vi "Main.vi"() -> ()   [LabVIEW 2014]
uses:
  Tasks.ctl
  <vilib>/Platform/TimedLoop/XDataNode/timing_clust.ctl
  <vilib>/Platform/TimedLoop/XDataNode/nitl_modes.ctl
  <vilib>/Platform/TimedLoop/XDataNode/wakeup.ctl
  <vilib>/myRIO/Instrument Drivers/Onboard IO/AI/typedefs/AI Reference.ctl
  <vilib>/myRIO/Common/Instrument Driver Framework/Utilities/typedefs/myRIO Generic Hardware Reference.ctl
  <vilib>/myRIO/Common/Instrument Driver Framework/Utilities/typedefs/Hardware Version Enum.ctl
  <vilib>/myRIO/Common/Instrument Driver Framework/Utilities/typedefs/myRIO v1.0 Reference.ctl
  <vilib>/myRIO/Common/Instrument Driver Framework/Utilities/typedefs/Generic FPGA Reference.ctl
  <vilib>/myRIO/Common/Instrument Driver Framework/myRIO v1.0/AI/typedefs/AI Channels List.ctl
  <vilib>/myRIO/Common/Instrument Driver Framework/myRIO v1.0/AI/typedefs/AI Channels Enum.ctl
  <vilib>/myRIO/Common/Instrument Driver Framework/Utilities/typedefs/Analog Scaling Constants List.ctl
  <vilib>/myRIO/Common/Instrument Driver Framework/Utilities/typedefs/Analog Scaling Constants.ctl
  <vilib>/userdefined/High Color/nirio_resource_hc.ctl
  <vilib>/myRIO/Common/Instrument Driver Framework/Utilities/vis/Is FPGA Ref Available.vi
  <vilib>/myRIO/Common/Instrument Driver Framework/myRIO v1.0/AI/vis/myRIO v1.1 Open Throughput AI.vi
  <vilib>/myRIO/Instrument Drivers/Onboard IO/AI/vis/Read.vi
  <vilib>/myRIO/Common/Instrument Driver Framework/Utilities/vis/Validate Channels.vi
  <vilib>/myRIO/Common/Instrument Driver Framework/myRIO v1.0/AI/vis/myRIO v1.0 Reserve AI.vi
  <vilib>/myRIO/Instrument Drivers/Onboard IO/DIO/vis/Write.vi
  <vilib>/myRIO/Instrument Drivers/Onboard IO/AO/vis/Write.vi
  <vilib>/myRIO/Common/Instrument Driver Framework/myRIO v1.0/UART/vis/myRIO v1.0 Close UART.vi
  <vilib>/myRIO/Common/Instrument Driver Framework/myRIO v1.0/AI/vis/myRIO v1.0 Build MUX Configuration AI.vi
  <vilib>/myRIO/Common/Instrument Driver Framework/myRIO v1.0/Resource Manager/vis/myRIO v1.0 Reserve Channel List.vi
  <vilib>/myRIO/Common/Instrument Driver Framework/myRIO v1.0/Resource Manager/vis/myRIO v1.0 Reserve Channel.vi
  <vilib>/myRIO/Common/Instrument Driver Framework/myRIO v1.0/Resource Manager/vis/myRIO v1.0 Unreserve Channel.vi
  <vilib>/myRIO/Common/Instrument Driver Framework/myRIO v1.0/Resource Manager/vis/myRIO v1.0 Build Mutex Name.vi
  <vilib>/Utility/VariantDataType/GetNumericInfo.vi
  <vilib>/Utility/error.llb/Error Cluster From Error Code.vi
  <vilib>/myRIO/Common/Instrument Driver Framework/myRIO v1.0/myRIO v1.1 Open Throughput.vi
  <vilib>/myRIO/Common/Instrument Driver Framework/myRIO v1.0/AI/vis/myRIO v1.0 Get Scaling Constants AI.vi
  <vilib>/myRIO/Common/Instrument Driver Framework/Utilities/vis/IO Manager.vi
  <vilib>/myRIO/Common/Instrument Driver Framework/Utilities/vis/Configuration Manager.vi
  <vilib>/myRIO/Common/Instrument Driver Framework/myRIO v1.0/myRIO v1.0 Close.vi
  <vilib>/myRIO/Common/Instrument Driver Framework/myRIO v1.0/AI/vis/myRIO v1.0 Read AI.vi
  <vilib>/functionblocks/Accumulate/Collect Numeric Array/Collect Numeric Array.vi
  <vilib>/myRIO/Instrument Drivers/Onboard IO/DIO/vis/Smart Open.vi
  <vilib>/myRIO/Common/Instrument Driver Framework/myRIO v1.0/DIO/vis/myRIO v1.0 Write DIO.vi
  <vilib>/myRIO/Instrument Drivers/Onboard IO/AO/vis/Smart Open.vi
  <vilib>/myRIO/Common/Instrument Driver Framework/myRIO v1.0/AO/vis/myRIO v1.0 Write AO.vi
  <vilib>/myRIO/Common/Instrument Driver Framework/Utilities/vis/FPGA Ref Manager.vi
  <vilib>/myRIO/Common/Instrument Driver Framework/myRIO v1.0/myRIO v1.0 Reset FPGA.vi
  <vilib>/myRIO/Common/Instrument Driver Framework/myRIO v1.0/IRQ/vis/myRIO v1.0 IRQ Info FGV.vi
  <vilib>/myRIO/Common/Instrument Driver Framework/myRIO v1.0/IRQ/vis/myRIO v1.0 Timer IRQ Info FGV.vi
  <vilib>/myRIO/Common/Instrument Driver Framework/myRIO v1.0/IRQ/vis/myRIO v1.0 ISR Agent.vi
  <vilib>/platform/TimedLoop/XDataNode/XDataNode.xnode
  <vilib>/myRIO/Express VI/Onboard IO/AI/AI Express VI.xnode
  <vilib>/myRIO/Instrument Drivers/Onboard IO/AI/vis/myRIO AI Open.xnode
  <vilib>/functionblocks/FB Core/FB Core.xnode
  <vilib>/myRIO/Instrument Drivers/Utilities/Utilities.lvlib
  <vilib>/Platform/TimedLoop/XDataNode/XDNodeRunTimeDep.lvlib
  <vilib>/myRIO/Instrument Drivers/Onboard IO/AI/AI.lvlib
  <vilib>/functionblocks/NI_FunctionBlock Libraries.lvlib
  <vilib>/ptbypt/NI_PtbyPt.lvlib
panel:
  in  "NPN2":dbl=5.0 format="%#_13g"
  in  "NPN1":dbl=5.0 format="%#_13g"
  out "LED1?":bool
  out "Stops":bool
  # "The myRIO Project template acquires acceleration data from the onboard accelerometer and displays the changes of acceleration values in a waveform chart."
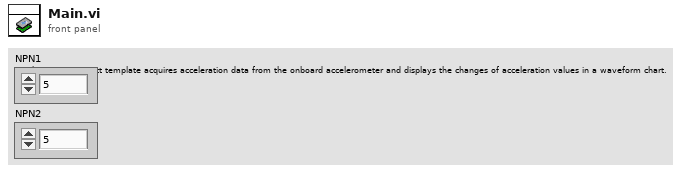
[diagram p1: front panel]
types:
  T1 = typedef "Tasks.ctl" = enum16{"Stop", "LEDs Off", "LED1 On", "LED2 On"}
  T2 = typedef "XDNodeRunTimeDep.lvlib/timing_clust.ctl" = cluster{"Expected End [f-1]":u64, "Actual End [f-1]":u64, "Finished Late? [f-1]":bool, "Expected End [i-1]":u64, "Actual End [i-1]":u64, "Finished Late? [i-1]":bool, "Expected Start [i]":u64, "Actual Start [i]":u64, "Expected Start [f]":u64, "Actual Start [f]":u64, "Source Name":string, "Structure Name":string, "Period":i64, "Deadline":i64, "Offset":i64, "Start":i64, "Priority":i32, "Timeout":i32, "Mode":T3, "Wakeup Reason":T4, "Error":errorcluster, "Source Type":string, "Secondary Source Type":string, "Global End Time":u64, "Global Start Time":u64, "Frame Duration":u64, "Iteration Duration":u64, "Assigned CPU":i32, "I/O Scan Engine Mode":u32}
  T3 = typedef "XDNodeRunTimeDep.lvlib/nitl_modes.ctl" = enum32{"No Change", "Process missed periods, maintain original phase", "Discard missed periods, maintain original phase", "Process missed periods, ignore original phase", "Discard missed periods, ignore original phase"}
  T4 = typedef "XDNodeRunTimeDep.lvlib/wakeup.ctl" = enum32{"Normal", "Aborted", "Asynchronous wakeup", "Timing source error", "Timed loop error", "Timeout"}
  T5 = typedef "AI.lvlib/AI Reference.ctl" = cluster{"myRIO Reference":T6, "AI Channels List":T10, "AI Scaling Constants List":T12}
  T6 = typedef "myRIO Generic Hardware Reference.ctl" = cluster{"myRIO Model":T7, "myRIO Hardware Reference":T8}
  T7 = typedef "Hardware Version Enum.ctl" = enum16{"Unknown", "myRIO-1900", "myRIO-1950"}
  T8 = typedef "myRIO v1.0 Reference.ctl" = cluster{"Generic FPGA Reference":T9, "Allow multiple opens":bool}
  T9 = typedef "Generic FPGA Reference.ctl" = refnum<k20>
  T10 = typedef "AI Channels List.ctl" = T11[]
  T11 = typedef "AI Channels Enum.ctl" = enum16{"Not Connected", "AudioIn/Left", "AudioIn/Right", "C/AI0", "C/AI1", "A/AI0", "A/AI1", "A/AI2", "A/AI3", "B/AI0", "B/AI1", "B/AI2", "B/AI3"}
  T12 = typedef "Analog Scaling Constants List.ctl" = T13[]
  T13 = typedef "Analog Scaling Constants.ctl" = cluster{"LSB Weight (Volts)":dbl, "Offset (Volts)":dbl, "Signed?":bool}
  T14 = typedef "nirio_resource_hc.ctl" = tag
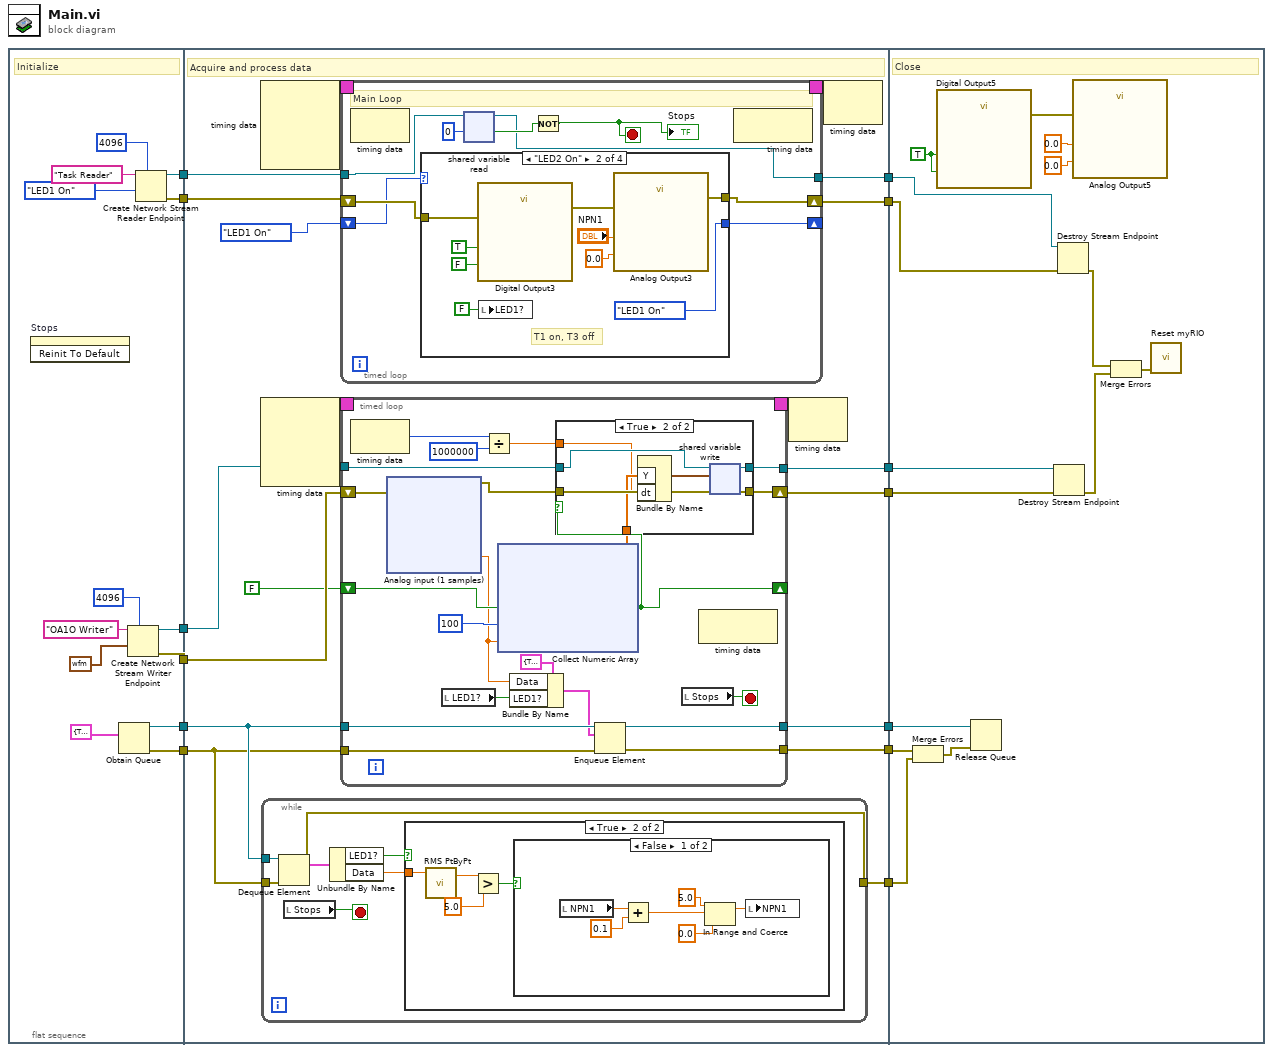
[diagram p0: block diagram]
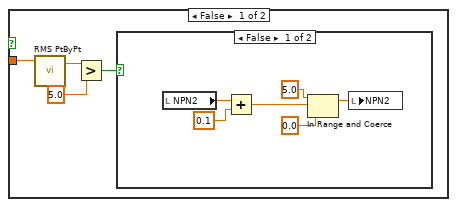
[diagram p2: hidden frame]
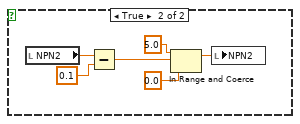
[diagram p3: hidden frame]
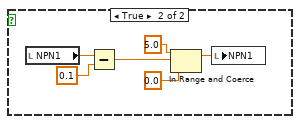
[diagram p4: hidden frame]
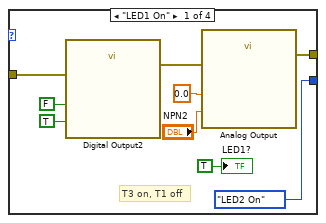
[diagram p5: hidden frame]
diagram:
  n1 = flat-sequence {
    tunnel: [w24] -> w13
    tunnel: [w23] -> w12
    tunnel: [w21] -> w9
    tunnel: [w20] -> w8
    tunnel: [w16] -> w5
    tunnel: [w15] -> w4
    tunnel: w13 -> [w45]
    tunnel: w12 -> [w44]
    tunnel: [w43] -> w11
    tunnel: [w42] -> w10
    tunnel: w9 -> [w39]
    tunnel: w8 -> [w40]
    tunnel: [w41] -> w7
    tunnel: [w38] -> w6
    tunnel: w5 -> [w29]
    tunnel: w4 -> [w28]
    tunnel: [w31] -> w3
    tunnel: [w30] -> w2
    tunnel: [w27] -> w1
    tunnel: w11 -> [w252]
    tunnel: w10 -> [w251]
    tunnel: w7 -> [w247]
    tunnel: w6 -> [w246]
    tunnel: w3 -> [w241]
    tunnel: w2 -> [w240]
    tunnel: w1 -> [w238]
    frame #0 {
      # "Initialize"
      n2 = invoke on="Stops" class="Bool (strict)" method="Reinit To Default"() -> ()  [unwired: 3 in, 3 out]
      n3 = Obtain Queue(element data type=cluster{"LED1?":bool, "Data":dbl} {"LED1?"=TRUE, "Data"=0.0}) -> (queue out=w16:refnum<queue>, error out=w15:errorcluster)  [unwired: 4 in, 1 out]
      n4 = Create Network Stream Writer Endpoint(7:4096 ("writer buffer size"), 9:waveform(dbl) {"t0"=timestamp(0 s since 1904-01-01), "dt"=1.0, "Y"=[]} ("output waveform"), 11:"OA1O Writer" ("writer name")) -> (0:w20:errorcluster, 3:w21:refnum<k21>)  [unwired: 4 in]
      n5 = Create Network Stream Reader Endpoint(7:4096 ("reader buffer size"), 9:Tasks."LED1 On" ("Tasks"), 11:"Task Reader" ("reader name")) -> (0:w23:errorcluster, 3:w24:refnum<k21>)  [unwired: 4 in]
    }
    frame #1 {
      # "Acquire and process data"
      n6 = node-c288() -> (w34:T2)  [unwired: 4 in]
      n7 = node-c288() -> (w36:T2)  [unwired: 4 in]
      n8 = while {
        tunnel: w29 -> [w52]
        tunnel: w28 -> [w51]
        tunnel: [w50] -> w27
        stop <- w48 stop-if-true
        n9 = Dequeue Element(queue=w52, error in (no error)=w51) -> (element=w49:cluster{"LED1?":bool, "Data":dbl}, error out=w50:errorcluster)  [unwired: 1 in, 2 out]
        n10 = local read "Stops"() -> (w48:bool)
        n11 = Unbundle By Name(w49) -> ("LED1?"=w47:bool, "Data"=w46:dbl)
        n12 = case shown="True" w47 {
          tunnel: w46 -> [w56 w72]
          frame False {
            n13 = call <vilib>:"RMS PtByPt.vi"("x"=w56) -> ("rms value"=w55:dbl)  [unwired: 3 in, 1 out]
            n14 = Greater?(x=w55, y=5.0) -> (0:w54:bool)
            n15 = case shown="False" w54 {
              frame False {
                n16 = local read "NPN2"() -> (w62:dbl)
                n17 = Add(x=w62, y=0.1) -> (x+y=w58:dbl)
                n18 = In Range and Coerce(upper limit=5.0, x=w58, lower limit=0.0) -> (coerced(x)=w59:dbl)  [unwired: 1 out]
                n19 = local write "NPN2"(w59) -> ()
              }
              frame True {
                n20 = local read "NPN2"() -> (w68:dbl)
                n21 = Subtract(x=w68, y=0.1) -> (x-y=w64:dbl)
                n22 = In Range and Coerce(upper limit=5.0, x=w64, lower limit=0.0) -> (coerced(x)=w65:dbl)  [unwired: 1 out]
                n23 = local write "NPN2"(w65) -> ()
              }
            }
          }
          frame True {
            n24 = call <vilib>:"RMS PtByPt.vi"("x"=w72) -> ("rms value"=w71:dbl)  [unwired: 3 in, 1 out]
            n25 = Greater?(x=w71, y=5.0) -> (0:w70:bool)
            n26 = case shown="False" w70 {
              frame False {
                n27 = local read "NPN1"() -> (w78:dbl)
                n28 = Add(x=w78, y=0.1) -> (x+y=w74:dbl)
                n29 = In Range and Coerce(upper limit=5.0, x=w74, lower limit=0.0) -> (coerced(x)=w75:dbl)  [unwired: 1 out]
                n30 = local write "NPN1"(w75) -> ()
              }
              frame True {
                n31 = local read "NPN1"() -> (w84:dbl)
                n32 = Subtract(x=w84, y=0.1) -> (x-y=w80:dbl)
                n33 = In Range and Coerce(upper limit=5.0, x=w80, lower limit=0.0) -> (coerced(x)=w81:dbl)  [unwired: 1 out]
                n34 = local write "NPN1"(w81) -> ()
              }
            }
          }
        }
      }
      n35 = timed-loop {
        tunnel: w45 -> [w86]
        tunnel: [w85] -> w42
        shift-right: [w92] -> w43
        shift-left: w44 -> [w93]
        timing: w34 -> [_]
        timing-out: [_] -> w33
        shift-right: [w90] -> _
        shift-left: Tasks."LED1 On" ("Tasks") -> [w91]
        stop <- w87 stop-if-true
        # "Main Loop"
        n36 = node-c288() -> ()  [unwired: 1 in, 1 out]
        n37 = case shown="\"LED2 On\"" w91 {
          tunnel: w93 -> [w97 w106 w112 w113]
          tunnel: [w96 w105 w112 w113] -> w92
          tunnel: [Tasks."LED2 On" ("Tasks") Tasks."LED1 On" ("Tasks") _ _] -> w90
          frame "LED1 On" {
            # "T3 on, T1 off"
            n38 = call "Digital Output2"("PNP1 (C/DIO0)"=FALSE, "PNP2 (C/DIO1)"=TRUE, "error in (no error)"=w97) -> ("error out"=w98:errorcluster)  [unwired: 24 in]
            n39 = call "Analog Output"("NPN1 (C/AO0)"=0.0, "NPN2 (C/AO1)"="NPN2", "error in (no error)"=w98) -> ("error out"=w96:errorcluster)  [unwired: 24 in]
            "LED1?" <- TRUE ("LED1?")
          }
          frame "LED2 On" {
            # "T1 on, T3 off"
            n40 = call "Digital Output3"("PNP1 (C/DIO0)"=TRUE, "PNP2 (C/DIO1)"=FALSE, "error in (no error)"=w106) -> ("error out"=w107:errorcluster)  [unwired: 24 in]
            n41 = local write "LED1?"(FALSE ("LED1?")) -> ()
            n42 = call "Analog Output3"("NPN1 (C/AO0)"="NPN1", "NPN2 (C/AO1)"=0.0, "error in (no error)"=w107) -> ("error out"=w105:errorcluster)  [unwired: 24 in]
          }
          frame "LEDs Off" {
          }
          frame "Stop" {
          }
        }
        n43 = shared-variable-read(w86, 0 ("timeout ms (-1)")) -> (w85:refnum<k21>, w88:bool)  [unwired: 1 in, 2 out]
        n44 = Not(x=w88) -> (.not. x?=w87:bool)
        "Stops" <- w87
        n45 = node-c288() -> ()  [unwired: 1 in, 1 out]
      }
      n46 = timed-loop {
        tunnel: w39 -> [w137]
        shift-right: [w130] -> w41
        shift-left: w40 -> [w135]
        tunnel: [w136] -> w38
        shift-right: [w131] -> _
        shift-left: FALSE ("full") -> [w132]
        timing: w36 -> [_]
        timing-out: [_] -> w35
        tunnel: w29 -> [w122]
        tunnel: w28 -> [w121]
        tunnel: [w120] -> w31
        tunnel: [w119] -> w30
        stop <- w138 stop-if-true
        n47 = node-c288() -> (w129:i64)  [unwired: 1 in]
        n48 = xnode "Analog input (1 samples)"("error in (no error)"=w135) -> ("OA1O (C/AI0 (AI0))"=w123:dbl, "error out"=w134:errorcluster)
        n49 = local read "LED1?"() -> (w125:bool)
        n50 = Divide(x=w129, y=i64 1000000) -> (x/y=w127:dbl)
        n51 = xnode "Collect Numeric Array"("reset"=w132, "array size"=u32 100, "input"=w123) -> ("full"=w131:bool, "collected data"=w124:dbl[])  [unwired: 1 in, 1 out]
        n52 = Bundle By Name(cluster=cluster{"LED1?":bool, "Data":dbl} {"LED1?"=TRUE, "Data"=0.0}, "Data"=w123, "LED1?"=w125) -> (w118:cluster{"LED1?":bool, "Data":dbl})
        n53 = case shown="True" w131 {
          tunnel: [w142 w150] -> w130
          tunnel: w137 -> [w143 w149]
          tunnel: [w143 w148] -> w136
          tunnel: w134 -> [w142 w147]
          tunnel: w124 -> [_ w146]
          tunnel: w127 -> [_ w145]
          frame False {
          }
          frame True {
            n54 = Bundle By Name("Y"=w146, "dt"=w145) -> (w144:waveform(dbl))  [unwired: 1 in]
            n55 = shared-variable-write(w149, w147, w144) -> (w148:refnum<k21>, w150:errorcluster)  [unwired: 1 in, 1 out]
          }
        }
        n56 = Enqueue Element(queue=w122, element=w118, error in (no error)=w121) -> (queue out=w120:refnum<queue>, error out=w119:errorcluster)  [unwired: 1 in, 1 out]
        n57 = local read "Stops"() -> (w138:bool)
        n58 = node-c288() -> ()  [unwired: 1 in, 1 out]
      }
      n59 = node-c288(w35) -> ()  [unwired: 1 out]
      n60 = node-c288(w33) -> ()  [unwired: 1 out]
    }
    frame #2 {
      w244 = TRUE ("PNP1 (C/DIO0)")
      # "Close"
      n61 = Merge Errors(w240, w238) -> (w239:errorcluster)
      n62 = call "Digital Output5"("PNP1 (C/DIO0)"=w244, "PNP2 (C/DIO1)"=w244) -> ("error out"=w245:errorcluster)  [unwired: 25 in]
      n63 = Release Queue(queue=w241, error in (no error)=w239) -> ()  [unwired: 1 in, 3 out]
      n64 = Destroy Stream Endpoint(8:w247, 11:w246) -> (0:w248:errorcluster)
      n65 = Destroy Stream Endpoint(8:w252, 11:w251) -> (0:w249:errorcluster)
      n66 = call "Analog Output5"("NPN1 (C/AO0)"=0.0, "NPN2 (C/AO1)"=0.0, "error in (no error)"=w245) -> ()  [unwired: 24 in, 1 out]
      n67 = Merge Errors(w249, w248) -> (w250:errorcluster)
      n68 = call <vilib>:"Reset myRIO.vi"("error in (no error)"=w250) -> ()  [unwired: 10 in, 1 out]
    }
  }
